vi "Subvi_Online_SVM_SWLDA.vi"(0 "rate":dbl=500.0 caption="Rate" format="%0.2f", 1 "Value":T1, 2 "Matrix":T1, 3 "in":T1, 5 "samples per channel":i32=25, 9 "Brain_data_source":dbl[](array[numeric]) caption="EEG_Raw_Data" format="%0.3f", 11 "Target_Flash_Order":i64[][](array[numeric])) -> (4 "output-0~8":i32, 6 "decision":dbl[](array[numeric]), 8 "ERP_발생여부":bool, 10 "SWLDA":dbl[](array[numeric]), 13 "EPR_발생_total":i16[](array[numeric]), 14 "ERP_all":dbl[][](array[numeric]), 15 "ERP_Parameters":dbl[][](array[numeric]))   [LabVIEW 2014]
uses:
  <vilib>/Analysis/Matrix/Datatypes/RealMatrix.ctl
  <vilib>/Analysis/3filter.llb/Filter Passband Type.ctl
  <vilib>/Analysis/baseanly.llb/Mean (DBL).vi
  <vilib>/Analysis/3filter.llb/Butterworth Filter (DBL).vi
  <vilib>/Utility/file.llb/Read From Spreadsheet File (DBL).vi
  <vilib>/Analysis/Matrix/Numeric/Conversions/Array To Matrix - RA.vi
  <vilib>/Analysis/Matrix/Numeric/Multiply/Multiply - RM,RM.vi
  <vilib>/Analysis/Matrix/Numeric/Subtract/Subtract - RM,RM.vi
  <vilib>/Analysis/Matrix/Numeric/Conversions/Matrix To Array - RM.vi
  <vilib>/Analysis/NI_AALBase.lvlib
  <vilib>/Analysis/Matrix/NI_Matrix.lvlib
panel:
  # "Input Values"
  # "Output Values"
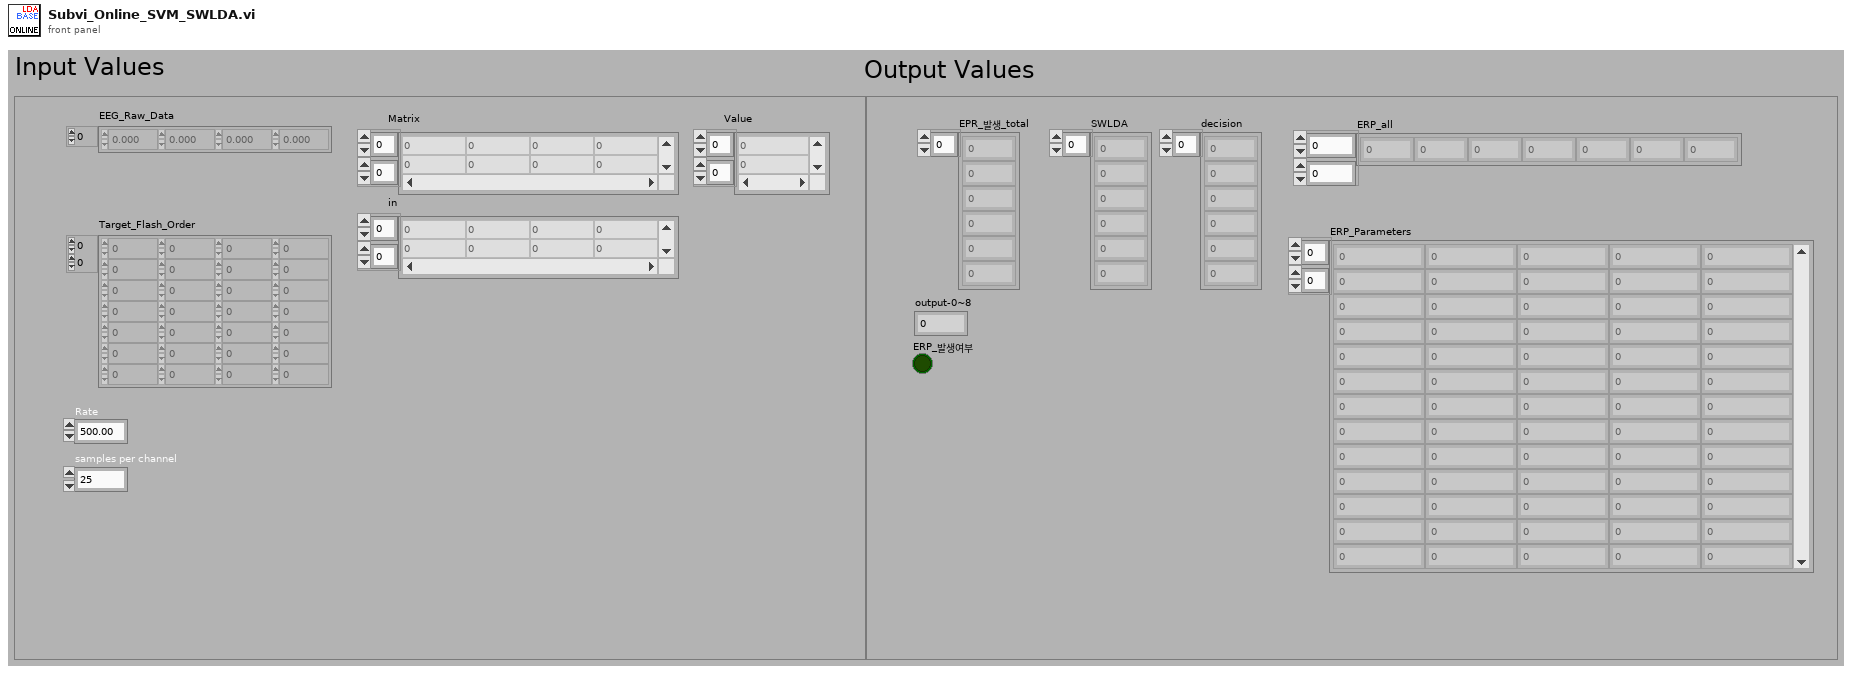
[diagram p1: front panel]
types:
  T1 = typedef "NI_Matrix.lvlib/RealMatrix.ctl" = dbl[][]
  T2 = typedef "NI_AALBase.lvlib/Filter Passband Type.ctl" = enum32{"Lowpass", "Highpass", "Bandpass", "Bandstop"}
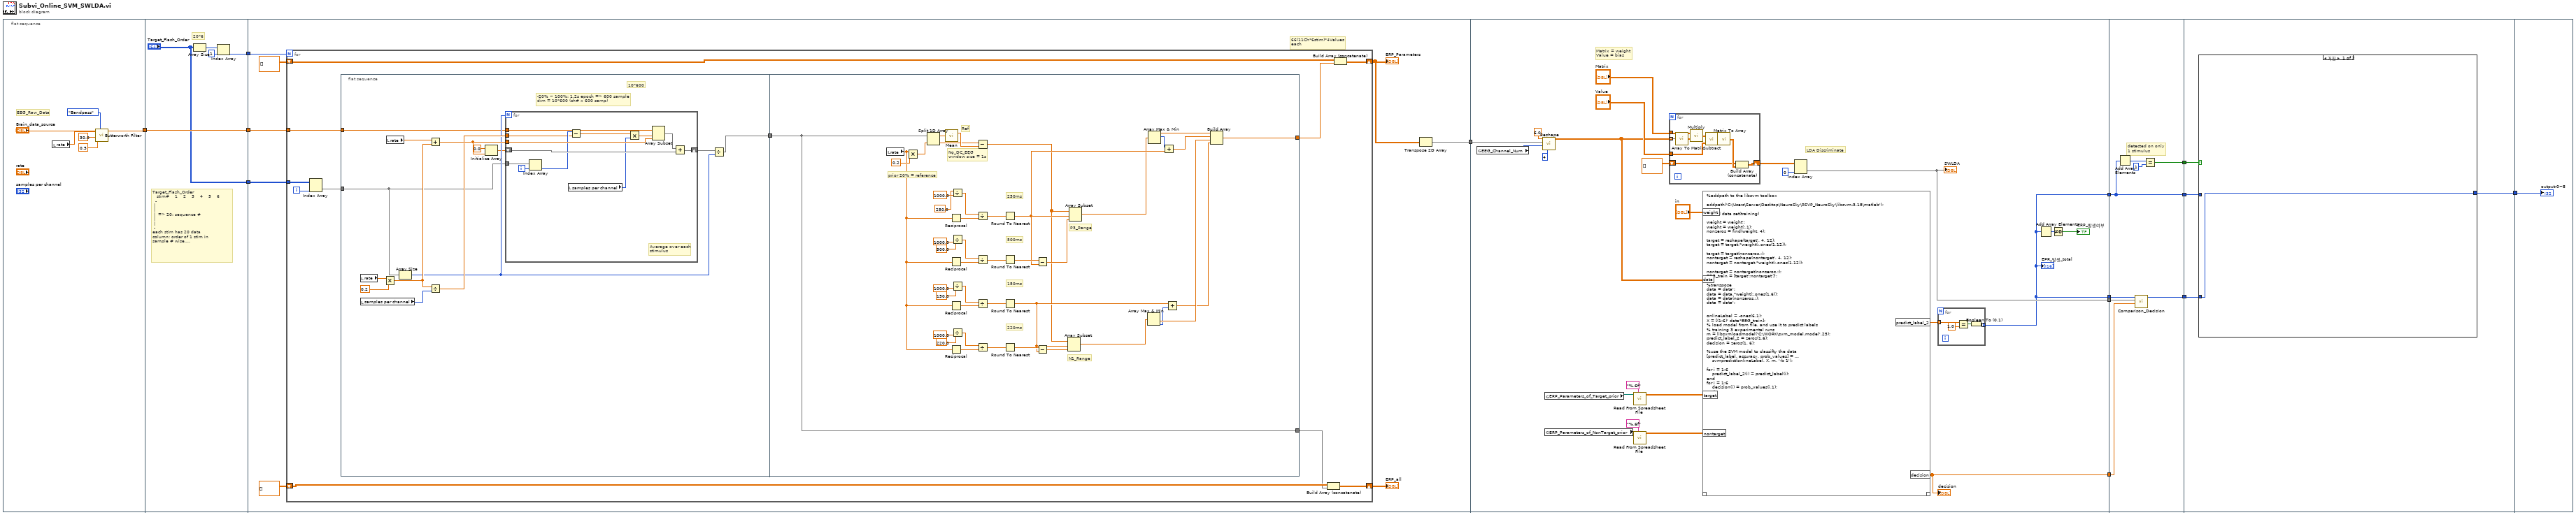
[diagram p0: block diagram]
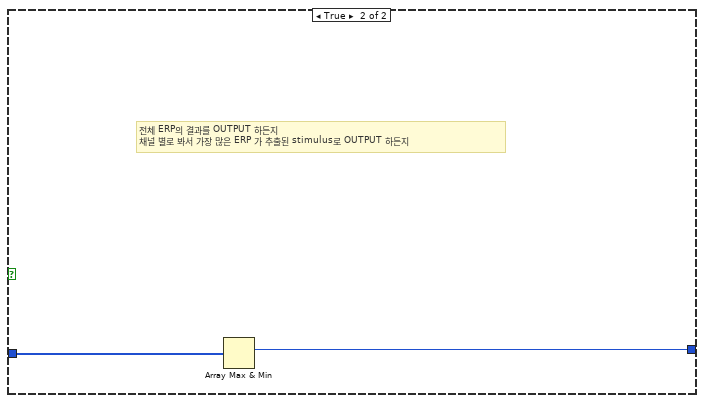
[diagram p2: hidden frame]
diagram:
  n1 = flat-sequence {
    tunnel: [w14] -> w13
    tunnel: [w24] -> w12
    tunnel: ["Target_Flash_Order"] -> w11
    tunnel: w13 -> [w24]
    tunnel: [w21] -> w10
    tunnel: w12 -> [w32]
    tunnel: w11 -> [w31]
    tunnel: w10 -> [w30]
    tunnel: [w27] -> w9
    tunnel: w9 -> [w122]
    tunnel: [w115] -> w8
    tunnel: [w115] -> w7
    tunnel: [w130] -> w5
    tunnel: [w116] -> w2
    tunnel: [w156] -> w4
    tunnel: [w155] -> w3
    tunnel: [w154] -> w1
    tunnel: w2 -> [w149]
    tunnel: w5 -> [w150]
    tunnel: w7 -> [w151]
    tunnel: w8 -> [w156]
    tunnel: [w160] -> w6
    tunnel: w4 -> [w158]
    tunnel: w3 -> [w159]
    tunnel: w1 -> [w157]
    tunnel: w6 -> [w164]
    frame #0 {
      # "EEG_Raw_Data"
      n2 = local read "rate"() -> (w16:dbl)
      n3 = call-poly <vilib>:"Butterworth Filter.vi"("filter type"=Filter_Passband_Type."Bandpass", "low cutoff freq: fl"=0.5, "high cutoff freq: fh"=30.0, "sampling freq: fs"=w16, "X"="Brain_data_source") -> ("Filtered X"=w14:dbl[])  [unwired: 3 in, 1 out]
    }
    frame #1 {
      # "Target_Flash_Order\n   stim#    1    2    3    4    5    6    \n  -\n |\n |\n |  => 20: sequence # \n |\n |\n -\neach stim has 20 data\ncolumn: order of 1 stim in \nsample # wise...."
      # "20*6"
      n4 = Array Size(array="Target_Flash_Order") -> (size(s)=w23:i32[])
      n5 = Index Array(array=w23, index=1 ("인덱스")) -> (element=w21:i32)
    }
    frame #2 {
      # "66(11Ch*6stim)*4Values\neach"
      n6 = for {
        N: w30 -> [_]
        tunnel: w32 -> [w42]
        tunnel: w31 -> [w41]
        shift-right: [w38] -> w28
        shift-left: dbl[][] [] -> [w37]
        shift-right: [w35] -> w25
        shift-left: dbl[][] [] -> [w34]
        i -> [w40]
        n7 = Index Array(array=w41, index (col)=w40) -> (element=w39:i64[])  [unwired: 1 in]
        n8 = flat-sequence {
          tunnel: w42 -> [w49]
          tunnel: w39 -> [w48]
          tunnel: [w44] -> w43
          tunnel: w43 -> [w71]
          tunnel: [w70] -> w36
          tunnel: [w71] -> w33
          frame #0 {
            # "-20% ~ 100%: 1.2s epoch => 600 sample\ndim = 10*600 (ch# x 600 samp)"
            # "10*600"
            n9 = local read "rate"() -> (w53:dbl)
            n10 = local read "samples per channel"() -> (w51:i32)
            n11 = Multiply(x=w53, y=0.2) -> (x*y=w57:dbl)
            n12 = local read "rate"() -> (w55:dbl)
            n13 = Array Size(array=w48) -> (size(s)=w50:i32)
            n14 = Add(x=w55, y=w57) -> (x+y=w56:dbl)
            n15 = Divide(x=w57, y=w51) -> (x/y=w54:dbl)
            n16 = Initialize Array(0.0 ("element"), w56) -> (w47:dbl[])
            n17 = for {
              N: w50 -> [_]
              tunnel: w49 -> [w69]
              shift-right: [w66] -> w45
              shift-left: w47 -> [w67]
              tunnel: w56 -> [w65]
              tunnel: w48 -> [w63]
              tunnel: w54 -> [w61]
              i -> [w64]
              # "Average over each\nstimulus"
              n18 = Index Array(array=w63, index=w64) -> (element=w62:i64)
              n19 = local read "samples per channel"() -> (w58:i32)
              n20 = Subtract(x=w62, y=w61) -> (x-y=w59:dbl)
              n21 = Multiply(x=w59, y=w58) -> (x*y=w60:dbl)
              n22 = Array Subset(array=w69, index=w60, length=w65) -> (w68:dbl[])
              n23 = Add(x=w68, y=w67) -> (x+y=w66:dbl[])
            }
            n24 = Divide(x=w45, y=w50) -> (x/y=w44:dbl[])
          }
          frame #1 {
            # "P3_Range"
            # "N1_Range"
            # "220ms"
            # "150ms"
            # "500ms"
            # "250ms"
            # "No_DC_EEG\nwindow size = 1s"
            # "Ref"
            # "prior 20% = reference"
            n25 = local read "rate"() -> (w85:dbl)
            n26 = Multiply(x=w85, y=0.2) -> (x*y=w107:dbl)
            n27 = Split 1D Array(array=w71, index=w107) -> (first subarray=w106:dbl[], second subarray=w102:dbl[])
            n28 = call-poly <vilib>:"Mean.vi"("X"=w106) -> ("mean"=w105:dbl)  [unwired: 1 out]
            n29 = Reciprocal(x=w85) -> (1/x=w101:dbl)
            n30 = Reciprocal(x=w85) -> (1/x=w100:dbl)
            n31 = Reciprocal(x=w85) -> (1/x=w99:dbl)
            n32 = Reciprocal(x=w85) -> (1/x=w98:dbl)
            n33 = Divide(x=250.0, y=1000.0) -> (x/y=w97:dbl)
            n34 = Divide(x=500.0, y=1000.0) -> (x/y=w96:dbl)
            n35 = Divide(x=150.0, y=1000.0) -> (x/y=w95:dbl)
            n36 = Divide(x=220.0, y=1000.0) -> (x/y=w94:dbl)
            n37 = Subtract(x=w102, y=w105) -> (x-y=w72:dbl[])
            n38 = Divide(x=w97, y=w101) -> (x/y=w84:dbl)
            n39 = Divide(x=w96, y=w100) -> (x/y=w83:dbl)
            n40 = Divide(x=w95, y=w99) -> (x/y=w82:dbl)
            n41 = Divide(x=w94, y=w98) -> (x/y=w81:dbl)
            n42 = Round To Nearest(number=w84) -> (nearest integer value=w75:dbl)
            n43 = Round To Nearest(number=w83) -> (nearest integer value=w80:dbl)
            n44 = Round To Nearest(number=w82) -> (nearest integer value=w77:dbl)
            n45 = Round To Nearest(number=w81) -> (nearest integer value=w79:dbl)
            n46 = Subtract(x=w80, y=w75) -> (x-y=w76:dbl)
            n47 = Subtract(x=w79, y=w77) -> (x-y=w78:dbl)
            n48 = Array Subset(array=w72, index=w77, length=w78) -> (w73:dbl[])
            n49 = Array Subset(array=w72, index=w75, length=w76) -> (w74:dbl[])
            n50 = Array Max & Min(array=w73) -> (min value=w110:dbl, min index (indices)=w103:i32)  [unwired: 2 out]
            n51 = Array Max & Min(array=w74) -> (max value=w112:dbl, max index (indices)=w104:i32)  [unwired: 2 out]
            n52 = Add(x=w104, y=w75) -> (x+y=w111:dbl)
            n53 = Add(x=w77, y=w103) -> (x+y=w109:dbl)
            n54 = Build Array(w112, w111, w110, w109) -> (w70:dbl[])
          }
        }
        n55 = Build Array (concatenate)(w34, w33) -> (w35:dbl[][])
        n56 = Build Array (concatenate)(w37, w36) -> (w38:dbl[][])
      }
      "ERP_Parameters" <- w28
      "ERP_all" <- w25
      n57 = Transpose 2D Array(2D array=w28) -> (transposed array=w27:dbl[][])
    }
    frame #3 {
      # "Matrix = weight\nValue = bias"
      # "LDA Discriminate"
      n58 = global read "Control_Panel_정리.vi" "EEG_Channel_Num"() -> (w121:i32)
      n59 = call "Reshape.vi"("Numeric"=4, "EEG_Channel_Num"=w121, "all rows"=w122, "Numeric 2"=6.0) -> ("Array"=w118:dbl[][])  [unwired: 7 in]
      n60 = global read "Control_Panel_정리.vi" "ERP_Parameters_of_Target_prior"() -> (w128:path)
      n61 = global read "Control_Panel_정리.vi" "ERP_Parameters_of_NonTarget_prior"() -> (w126:path)
      n62 = call-poly <vilib>:"Read From Spreadsheet File.vi"("format (%.3f)"="%.6f", "file path (dialog if empty)"=w128) -> ("all rows"=w125:dbl[][])  [unwired: 5 in, 4 out]
      n63 = call-poly <vilib>:"Read From Spreadsheet File.vi"("format (%.3f)"="%.6f", "file path (dialog if empty)"=w126) -> ("all rows"=w124:dbl[][])  [unwired: 5 in, 4 out]
      n64 = for {
        tunnel: "Matrix" -> [w140]
        tunnel: "Value" -> [w146]
        shift-right: [w143] -> w133
        shift-left: dbl[][] [] -> [w142]
        tunnel: w118 -> [w141] mode=indexing
        n65 = call-poly <vilib>:"Array To Matrix.vi"("Real 1D Array"=w141) -> ("Real Matrix (Column Vector)"=w145:T1)
        n66 = call-poly <vilib>:"Multiply.vi"("Real Matrix B"=w145, "Real Matrix A"=w140) -> ("A * B"=w148:T1)
        n67 = call-poly <vilib>:"Subtract.vi"("Real Matrix B"=w146, "Real Matrix A"=w148) -> ("A - B"=w147:T1)
        n68 = call-poly <vilib>:"Matrix To Array.vi"("Real Matrix"=w147) -> ("Real 2D Array"=w144:dbl[][])
        n69 = Build Array (concatenate)(w142, w144) -> (w143:dbl[][])
      }
      n70 = script code="%addpath to the libsvm toolbox\n\naddpath('C:\\Users\\Server\\Desktop\\NeuroSky\\RSVP_NeuroSky\\libsvm-3.18\\matlab');\n\n%read data set(training)\n\nweight = weight';\nweight = weight(:,1);\nnonzeros = find(weight, 4);\n\ntarget = reshape(target', 4, 12);\ntarget = target.*weight(:,ones(1,12));\n\ntarget = target(nonzeros,:);\nnontarget = reshape(nontarget', 4, 12);\nnontarget = nontarget.*weight(:,ones(1,12));\n\nnontarget = nontarget(nonzeros,:);\nEEG_train = [target';nontarget']';\n\n%transpose\ndata = data';\ndata = data.*weight(:,ones(1,6));\ndata = data(nonzeros,:);\ndata = data';\n\n\nonlineLabel = -ones(6,1);\nX = [(1:6)' data*EEG_train];\n% load model from file, and use it to predict labels\n% training 3 experimental runs\nm = libsvmloadmodel('C:\\WORK\\svm_model.model',25);\npredict_label_2 = zeros(1,6);\ndecision = zeros(1, 6);\n\n%use the SVM model to classifty the data\n[predict_label, accuracy, prob_values] = ...\n    svmpredict(onlineLabel, X, m, '-b 1');\n\nfor i = 1:6\n    predict_label_2(i) = predict_label(i);\nend\nfor i = 1:6\n    decision(i) = prob_values(i,1);\nend"("weight"="in", "target"=w125, "nontarget"=w124, "data"=w118) -> ("predict_label_2"=w123:dbl[], "decision"=w116:dbl[])  [unwired: 1 in, 1 out]
      "decision" <- w116
      n71 = Index Array(array=w133, index (col)=0 ("비활성화된 인덱스 (열)")) -> (element=w130:dbl[])  [unwired: 1 in]
      "SWLDA" <- w130
      n72 = for {
        tunnel: w123 -> [w139] mode=indexing
        tunnel: [w138] -> w115 mode=indexing
        n73 = Equal?(x=w139, y=1.0) -> (x = y?=w136:bool)
        n74 = Boolean To (0,1)(Boolean=w136) -> (0, 1=w138:i16)
      }
      "EPR_발생_total" <- w115
      n75 = Add Array Elements(numeric array=w115) -> (sum=w114:i16)
      n76 = Not Equal To 0?(x=w114) -> (x != 0?=→"ERP_발생여부":bool)
    }
    frame #4 {
      # "detected on only\n1 stimulus"
      n77 = Add Array Elements(numeric array=w156) -> (sum=w153:i16)
      n78 = call "Comparison_Decision.vi"("decision"=w149, "SWLDA"=w150, "EPR_발생_total"=w151) -> ("selected"=w154:i32)  [unwired: 8 in]
      n79 = Equal?(x=w153, y=i16 1) -> (x = y?=w155:bool)
    }
    frame #5 {
      n80 = case shown="거짓" w159 {
        tunnel: [w161 w163] -> w160
        tunnel: w158 -> [_ w162]
        tunnel: w157 -> [w161 _]
        frame False {
        }
        frame True {
          # "전체 ERP의 결과를 OUTPUT 하든지\n채널 별로 봐서 가장 많은 ERP 가 추출된 stimulus로 OUTPUT 하든지"
          n81 = Array Max & Min(array=w162) -> (max index (indices)=w163:i32)  [unwired: 3 out]
        }
      }
    }
    frame #6 {
      "output-0~8" <- w164
    }
  }
